vi "FYP_VI_MIDI_Close.vi"(7 "midiOut":i32) -> (0 "midiOutClose Error Code":i32)   [LabVIEW 2013]
uses:
  winmm.dll
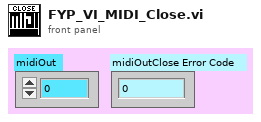
[diagram p1: front panel]
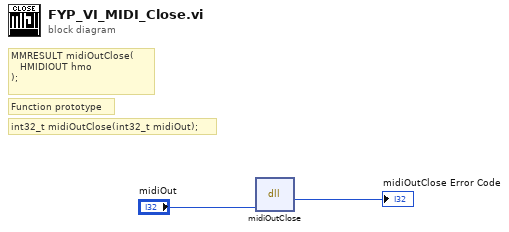
[diagram p0: block diagram]
diagram:
  # "MMRESULT midiOutClose(\n   HMIDIOUT hmo\n);"
  # "Function prototype"
  # "int32_t midiOutClose(int32_t midiOut);"
  n1 = dll-call lib="winmm.dll" fn="midiOutClose"("midiOut"="midiOut") -> ("return type"=→"midiOutClose Error Code":i32)  [unwired: 4 in, 2 out]
